vi "溶解氧电极校准.vi"() -> ()   [LabVIEW 2016, in "斯坦道多参数.lvlib"]
uses:
  <vilib>/Utility/miscctls.llb/LVPointTypeDef.ctl
  <vilib>/Analysis/NI_AALBase.lvlib
panel:
  out "标液2":string="饱和标准液"
  out "标液1":string="零点标准液"
  in  "刷新按钮":bool
  out "第二点信号值":dbl
  out "第一点信号值":dbl
  out "通讯状态":string
  out "第二点校准值":dbl
  out "第一点校准值":dbl
  out "最小值":sgl format="%#.2f"
  out "最大值":sgl format="%#.2f"
  in  "校准模式":u16(ring)=1 items=["两点校准", "单点校准"]
  in  "校准停止":bool
  in  "校准启动":bool
  out "波形图表":dbl(graph) caption="历史曲线"
  out "变异系数":dbl format="%#.6f"
  out "standard deviation":dbl caption="标准差" format="%#.2f"
  out "mean":dbl caption="均值" format="%#.2f"
  out "测量读值":dbl caption="测量值" format="%#.2f"
  out "偏移值补偿":dbl caption="溶解氧偏移修正值" format="%#.2f"
  out "饱和度值":dbl format="%#.2f"
  out "提示":string
  out "气压补偿值":dbl format="%#.2f"
  out "盐度补偿值":dbl format="%#.2f"
  out "电极斜率":dbl format="%#.6f"
  out "电极零点":dbl format="%#.6f"
  # "溶解氧电极设定"
  # "%"
  # "%"
  # "ppt"
  # "hPa"
  # "请选择校准模式:"
  # "mg/L"
  # "%"
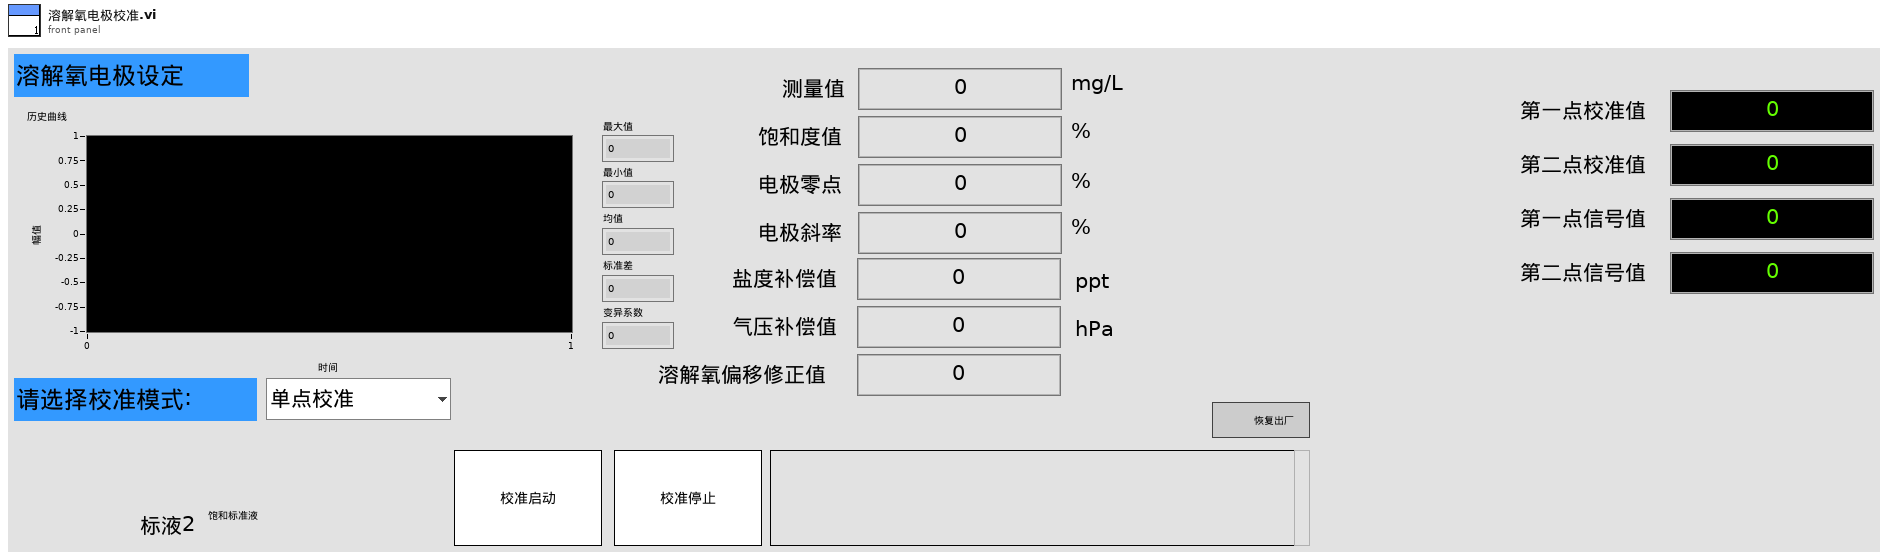
[diagram p1: front panel]
types:
  T1 = typedef "LVPointTypeDef.ctl" = cluster{"Horizontal":i16, "Vertical":i16}
  T2 = cluster{"电极状态标志":u16, "电极型号标志":u16, "溶解氧测量值":sgl, "温度测量值":sgl, "溶解氧饱和度值":sgl, "盐度补偿值":sgl, "大气压补偿值":sgl, "溶解氧偏移修正值":sgl, "温度偏移修正值":sgl, "手动温度补偿值":sgl, "溶解氧电极零点":sgl, "溶解氧电极斜率":sgl, "第1点标准值记录":sgl, "第1点信号值记录":sgl, "第1点温度值记录":sgl, "第2点标准值记录":sgl, "第2点信号值记录":sgl, "第2点温度值记录":sgl, "命令滤波设定":u16, "温度模式":enum16{"ATC", "MTC"}, "生产批次":u16, "电极序号":u16, "串口地址":u16, "串口波特率":enum16{"9600", "19200", "115200"}, "串口校验位":enum16{"NONE", "ODD", "EVEN"}, "串口停止位":enum16{"1bit", "2bit"}, "第一点标准值":sgl, "第二点标准值":sgl}
  T3 = enum8{"Enabled", "Disabled", "Disabled and Grayed Out"}
  T4 = cluster{"ph":bool, "DO":bool, "Cond":bool, "Turb":bool, "叶绿素a":bool, "藻密度":bool, "ORP":bool}
  T5 = cluster{"温度测量值":sgl, "测量值":sgl, "温度偏移修正值":sgl, "信号值":sgl}
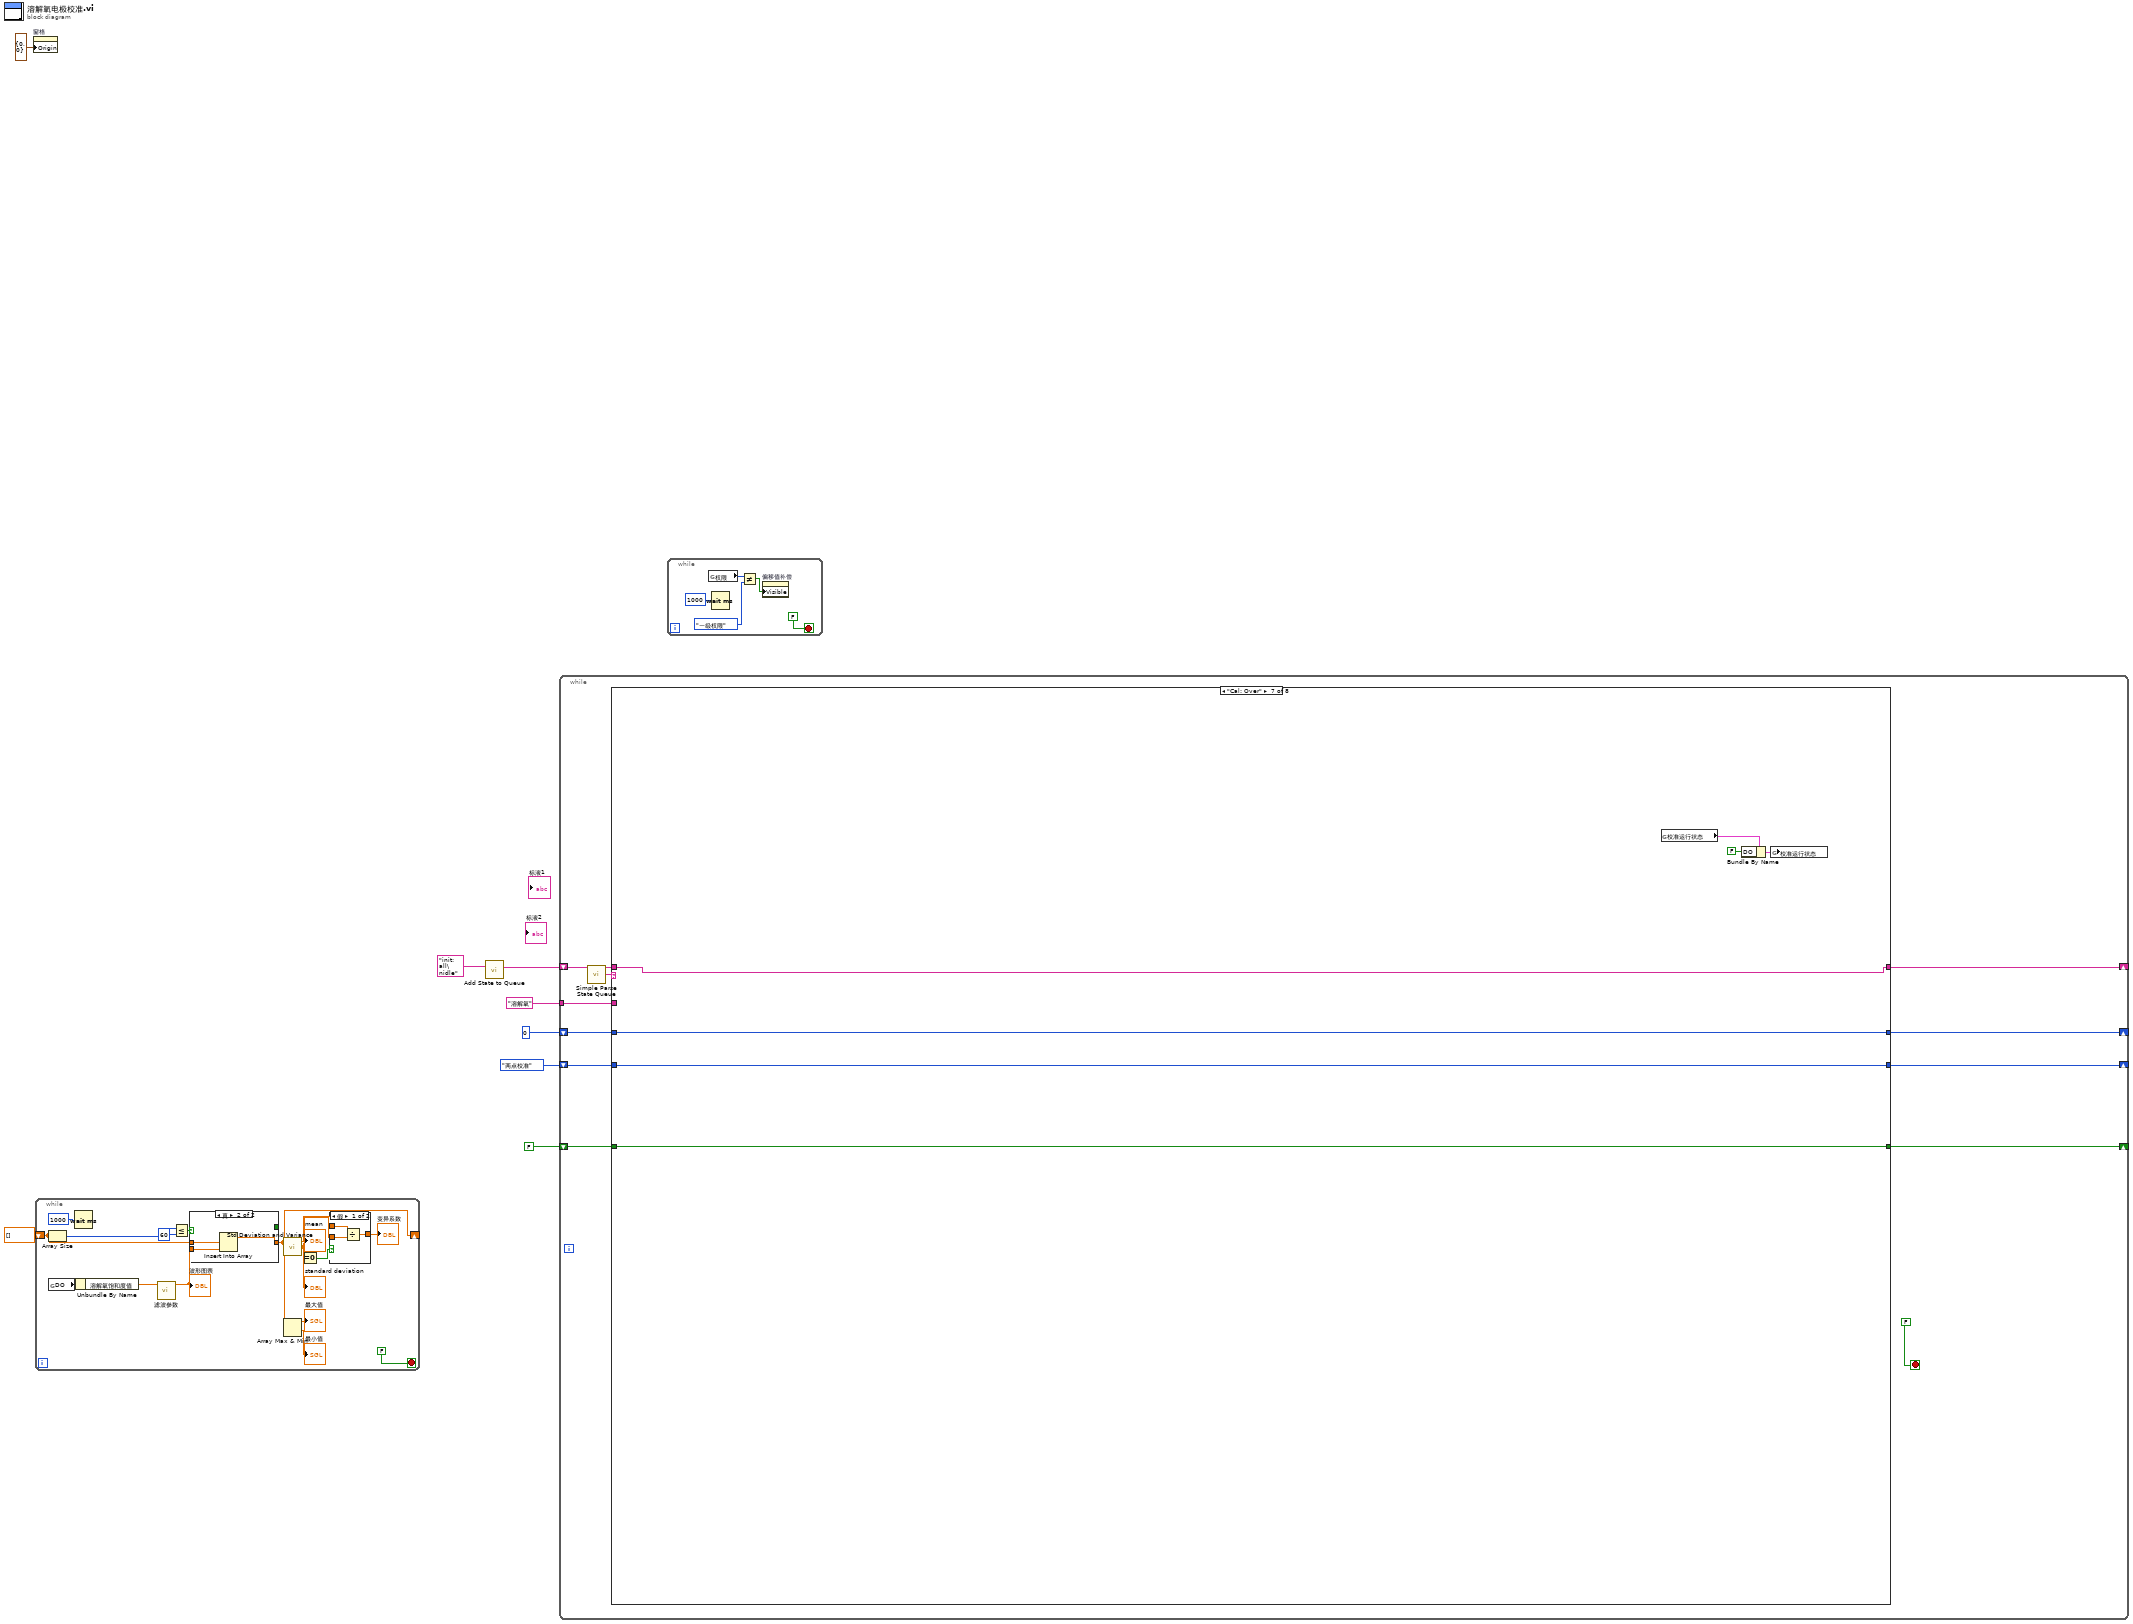
[diagram p0: block diagram]
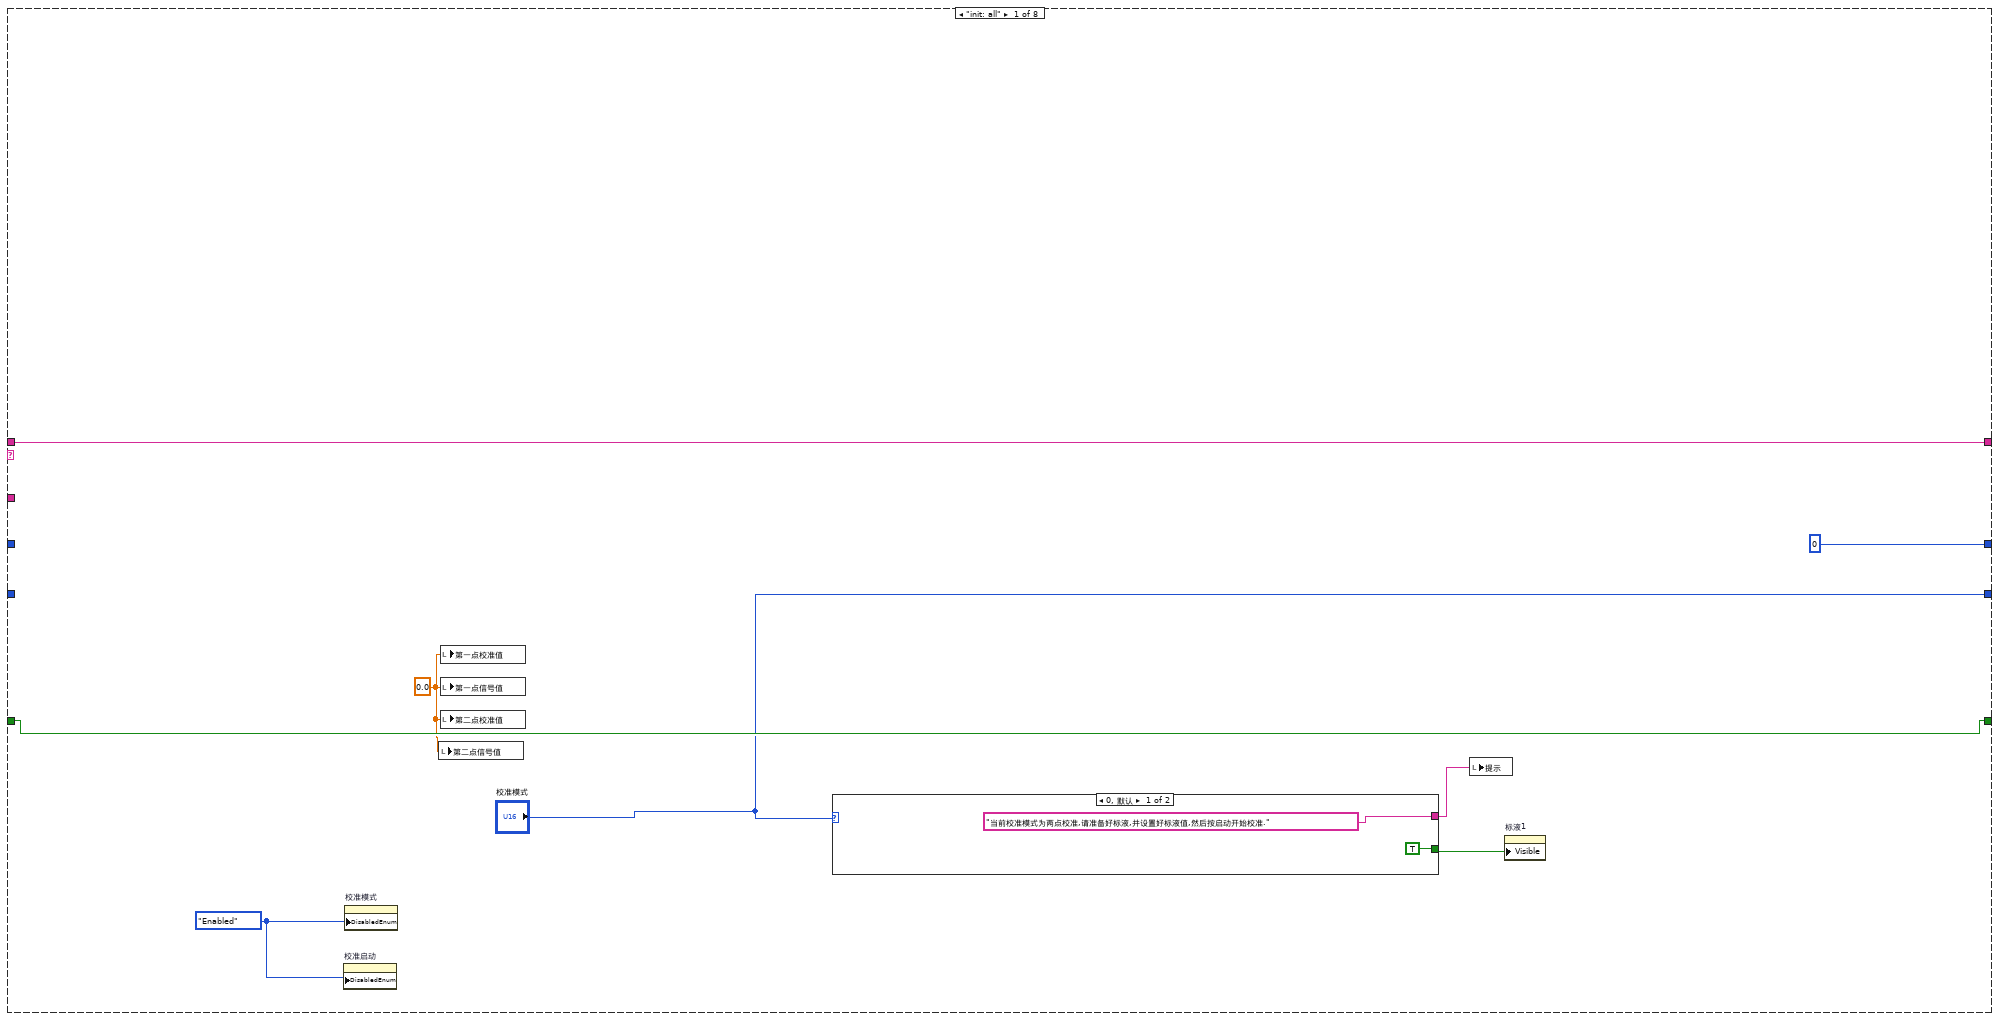
[diagram p2: hidden frame]
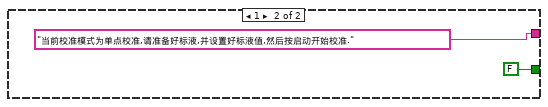
[diagram p3: hidden frame]
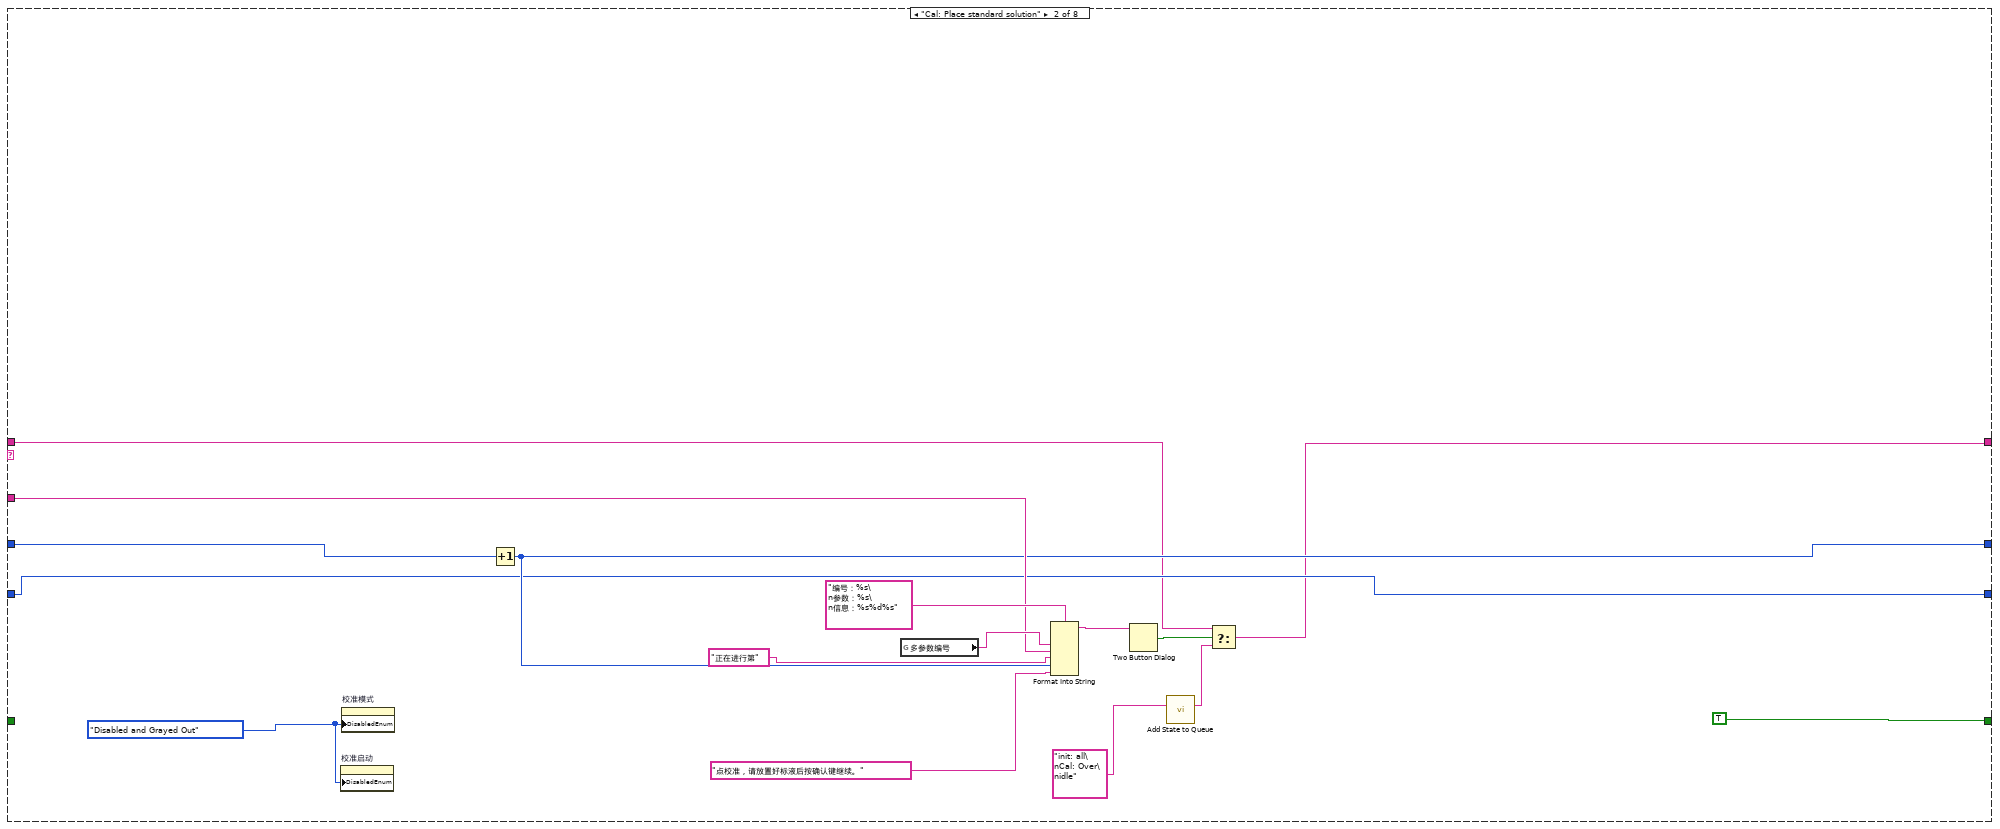
[diagram p4: hidden frame]
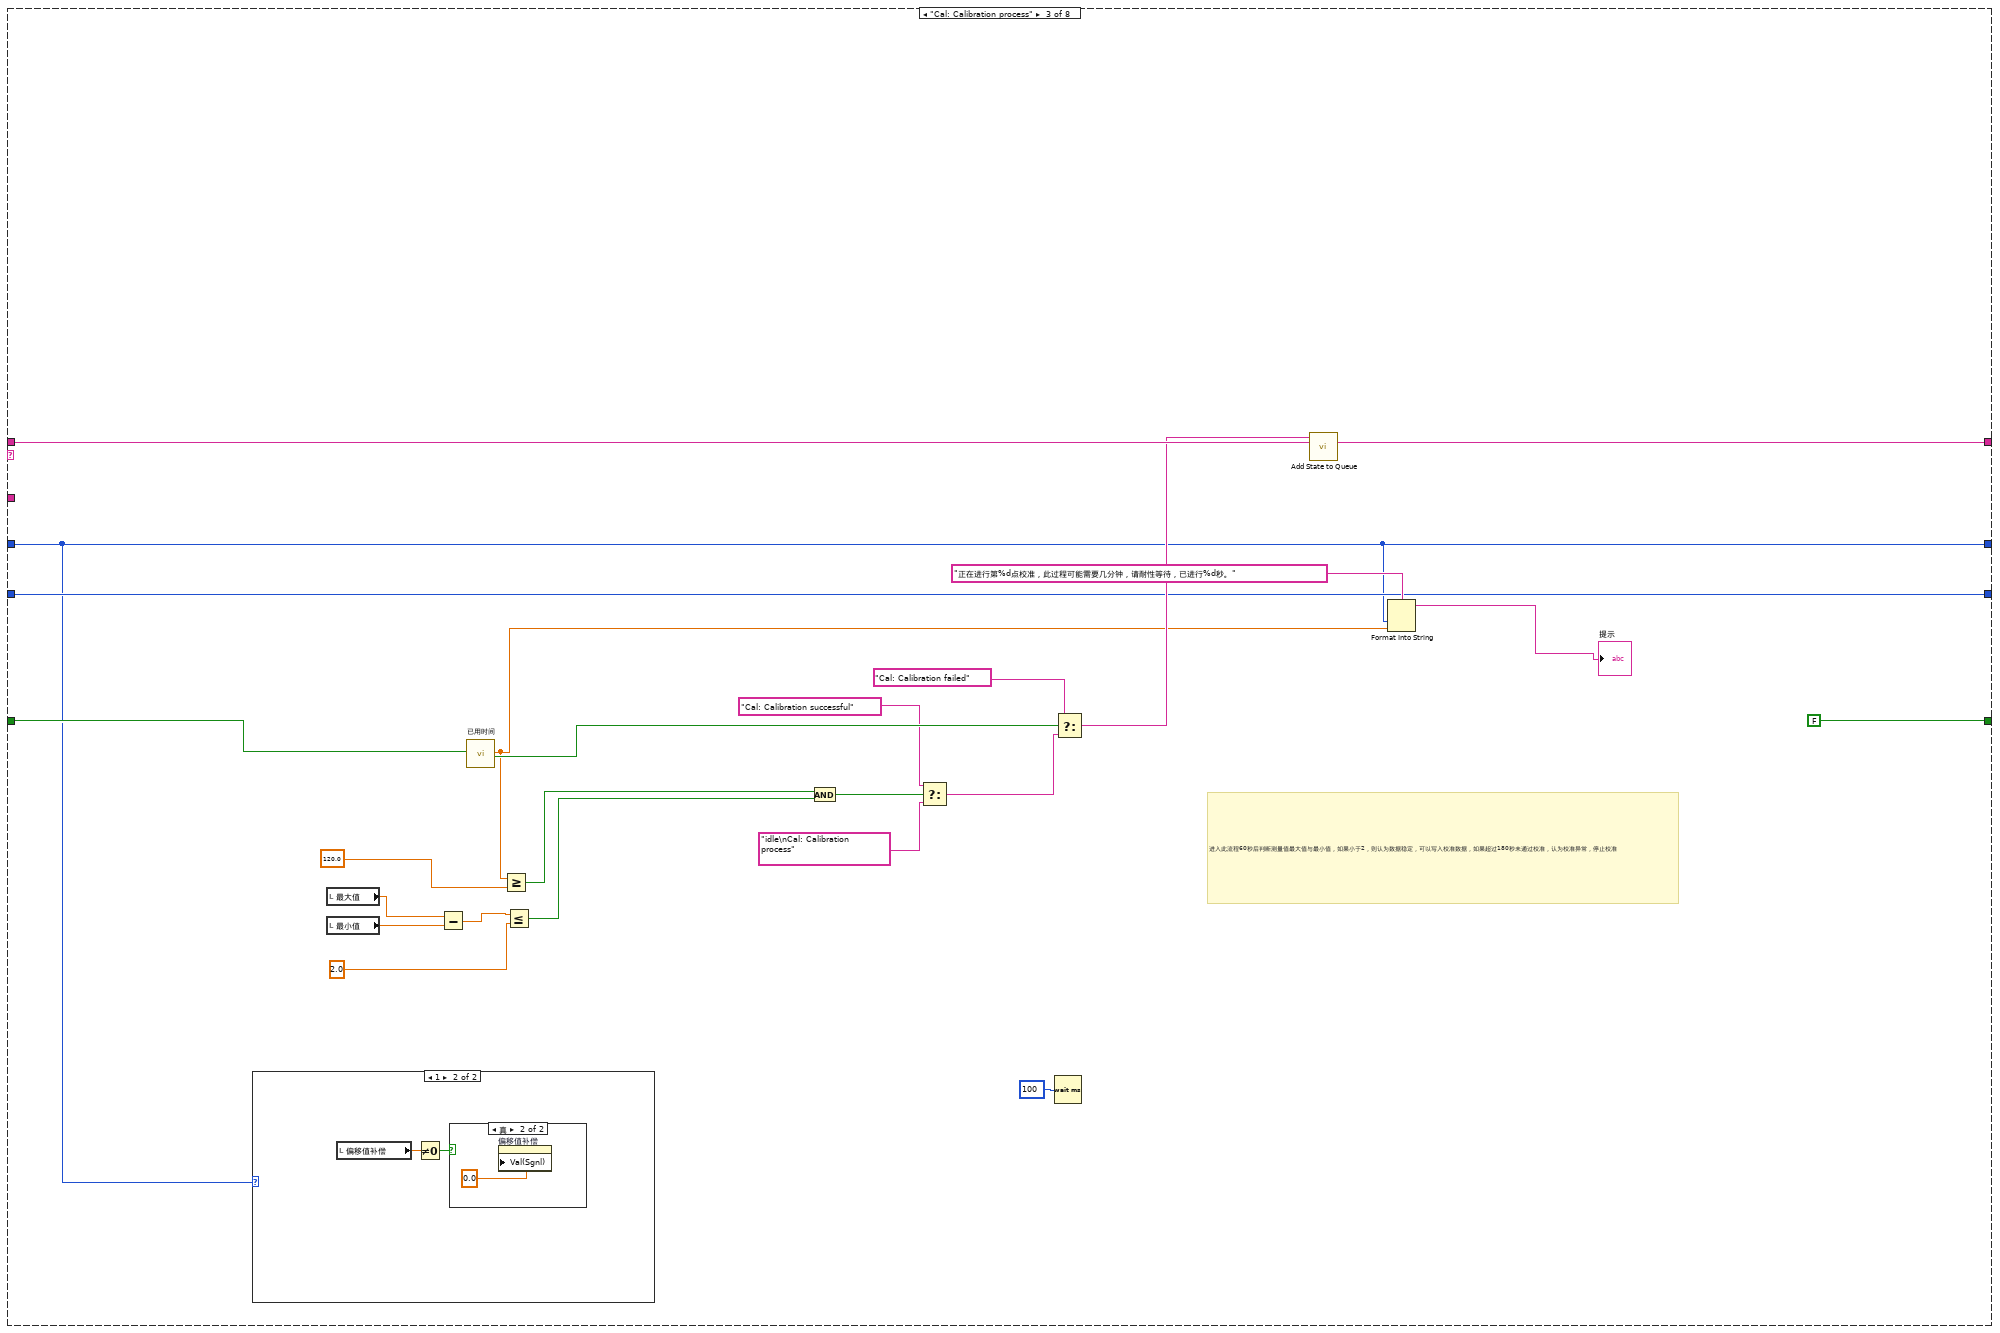
[diagram p5: hidden frame]
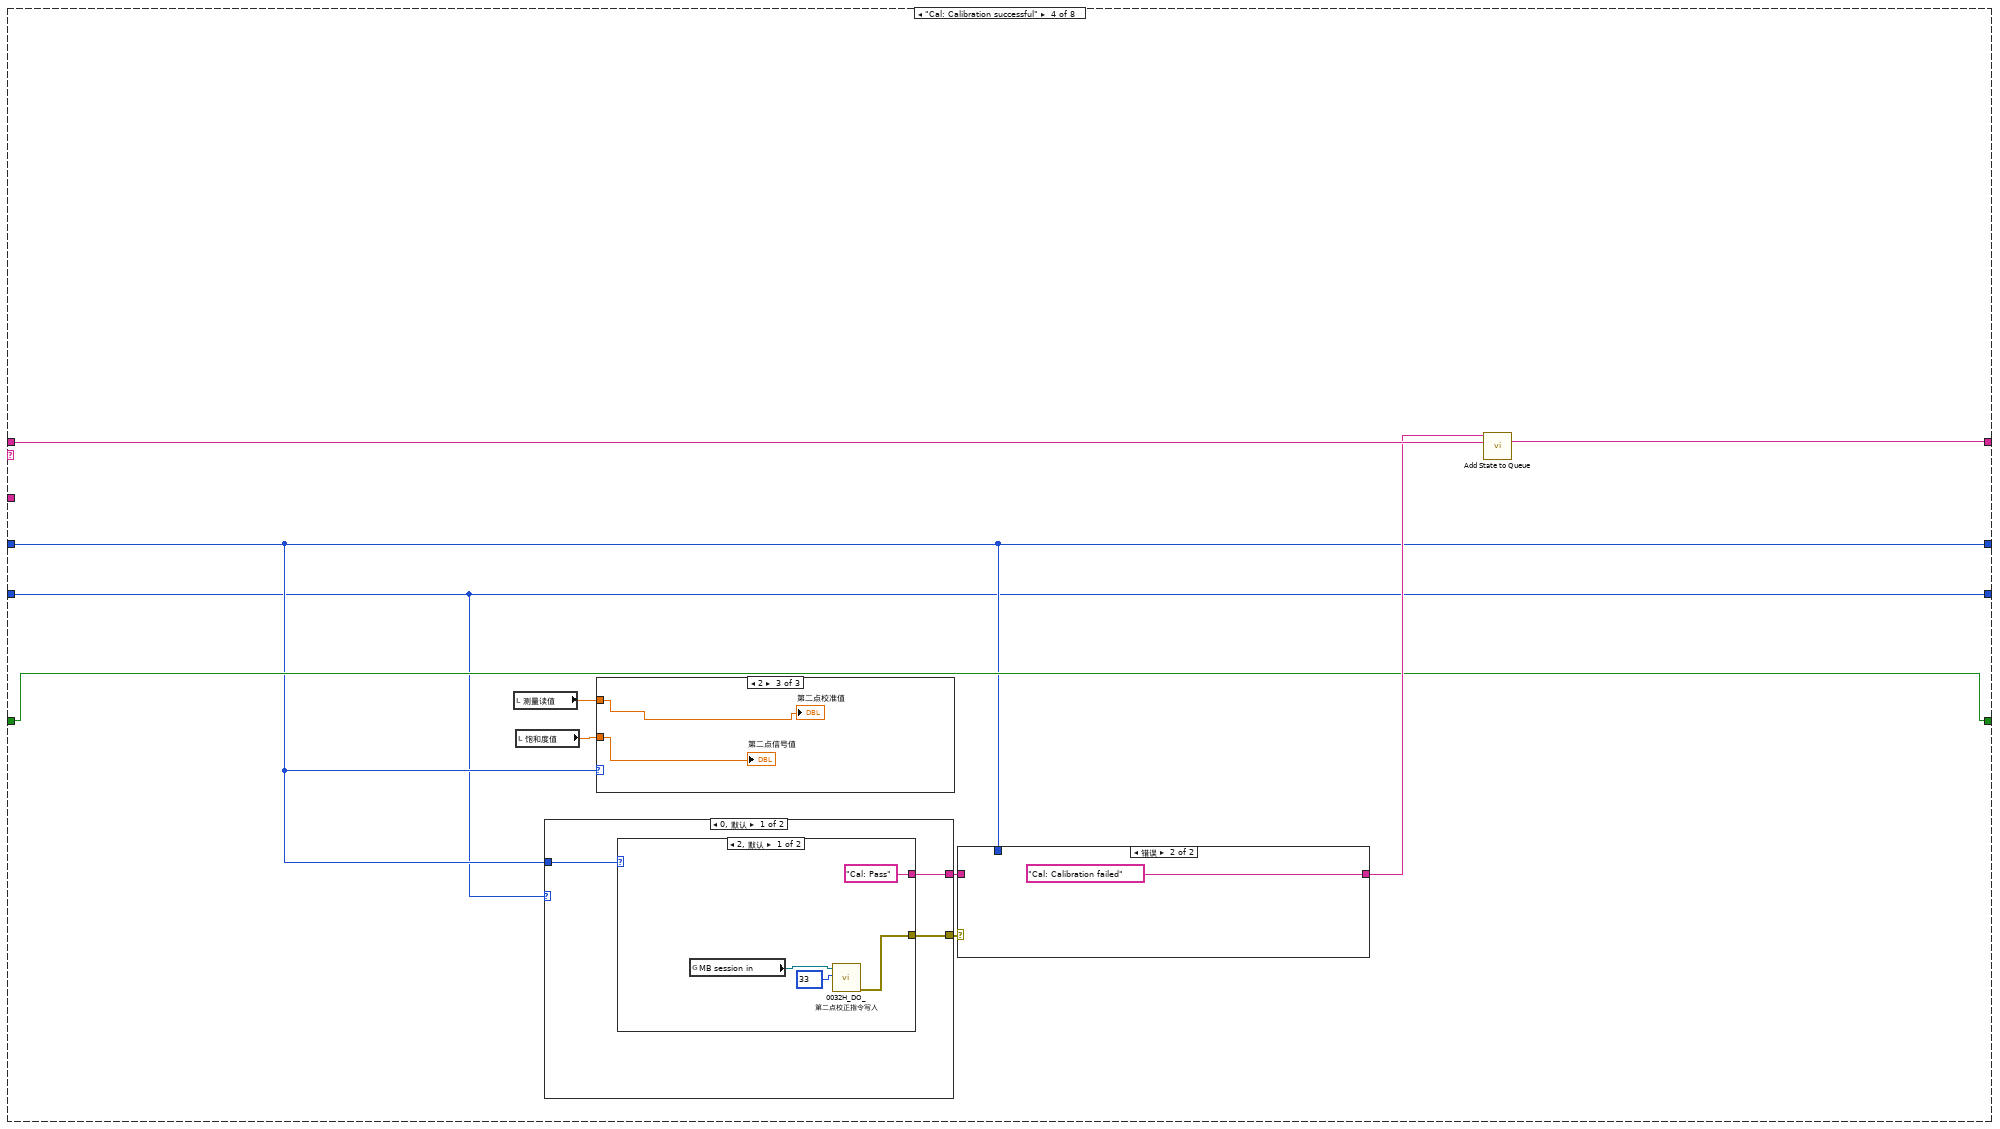
[diagram p8: hidden frame]
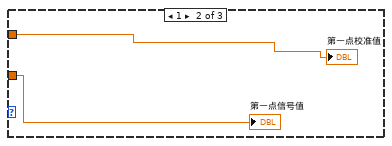
[diagram p10: hidden frame]
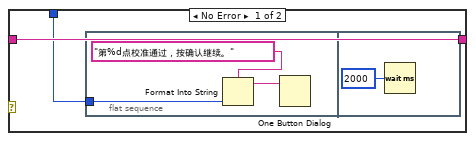
[diagram p11: hidden frame]
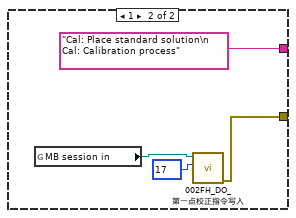
[diagram p12: hidden frame]
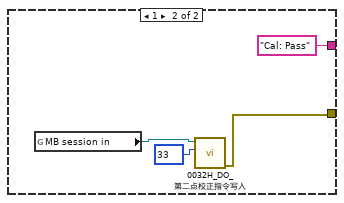
[diagram p13: hidden frame]
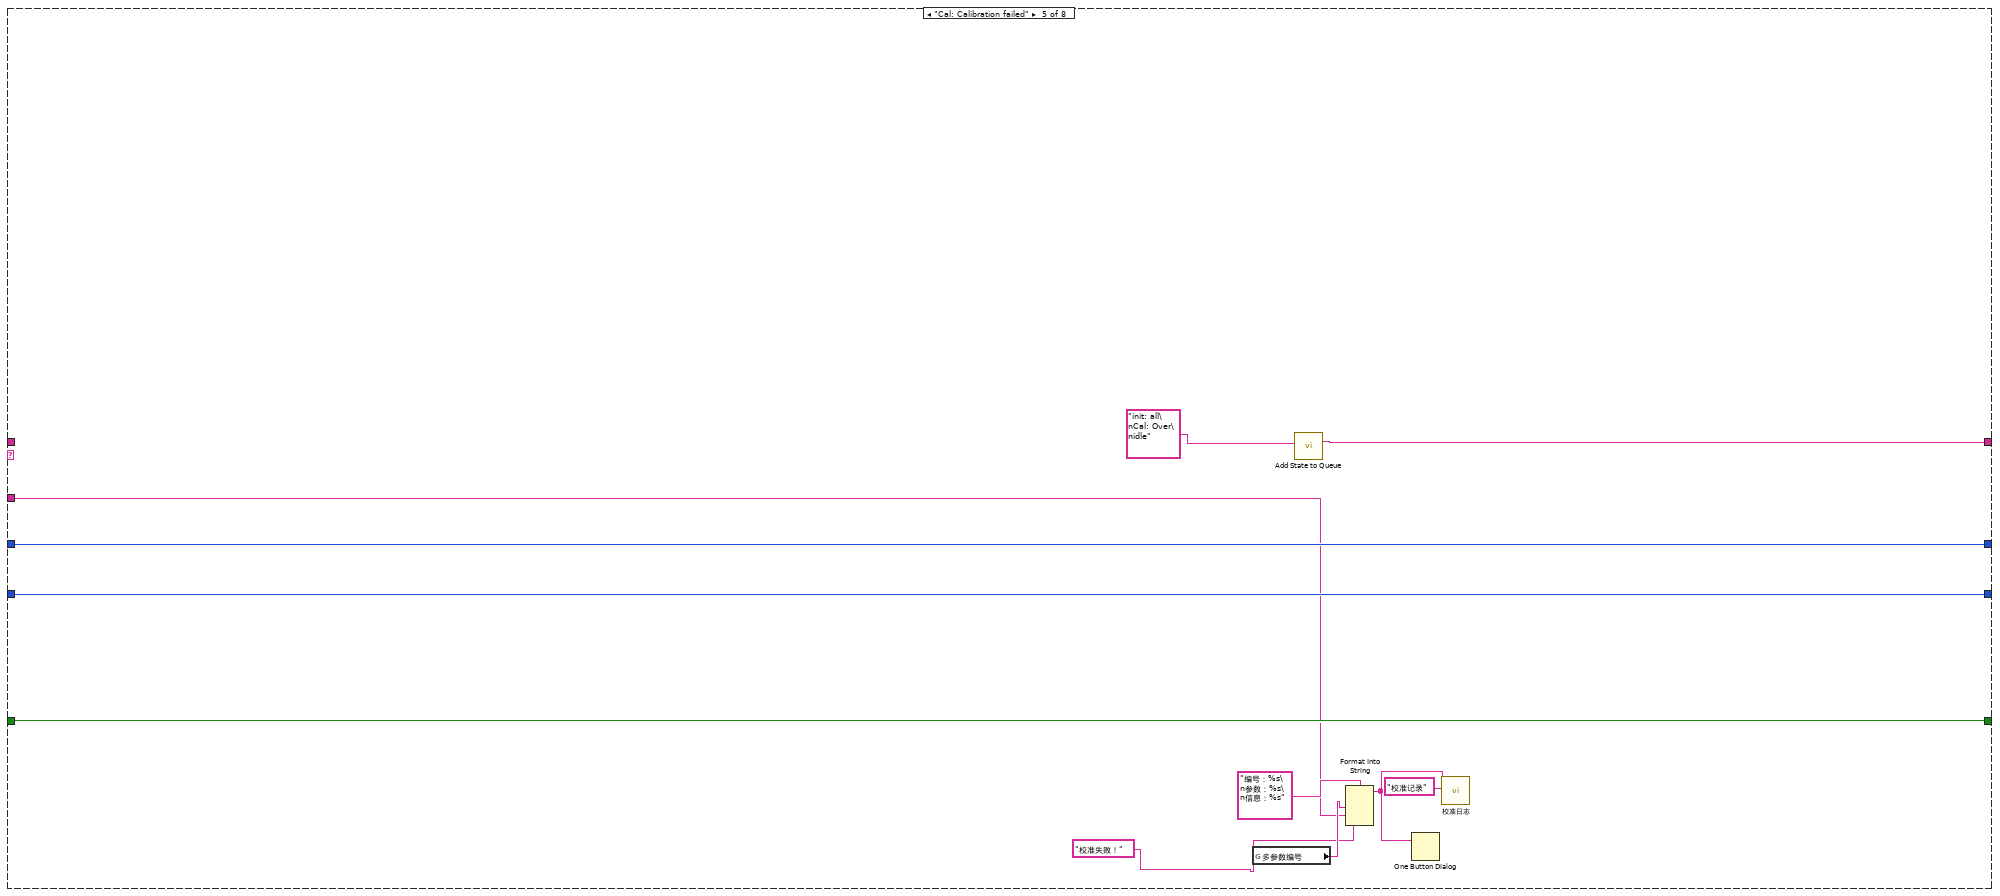
[diagram p14: hidden frame]
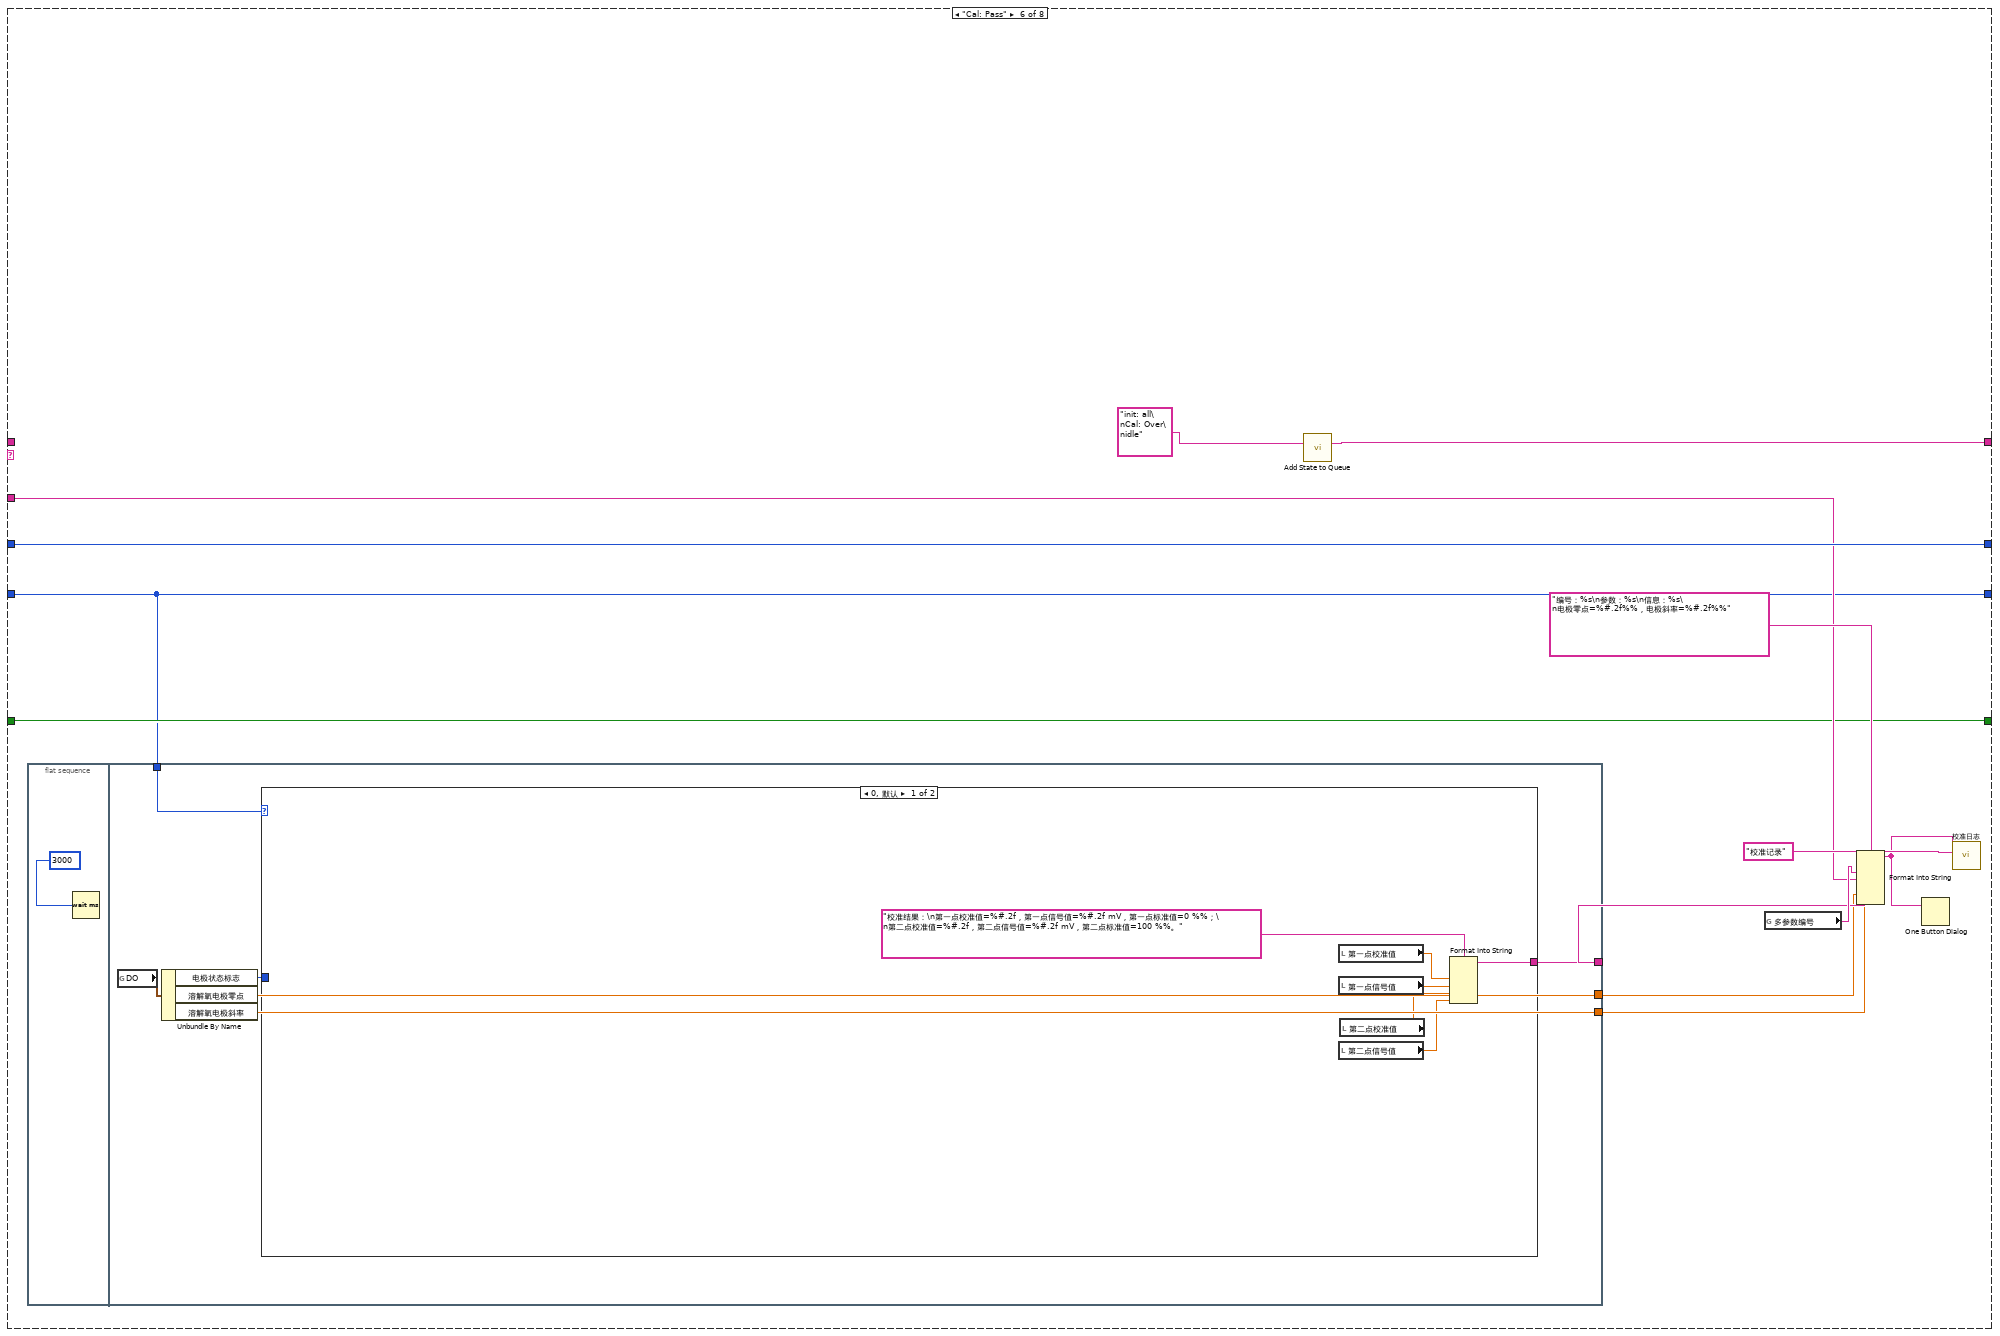
[diagram p15: hidden frame]
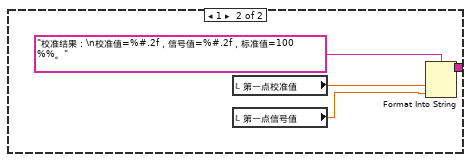
[diagram p16: hidden frame]
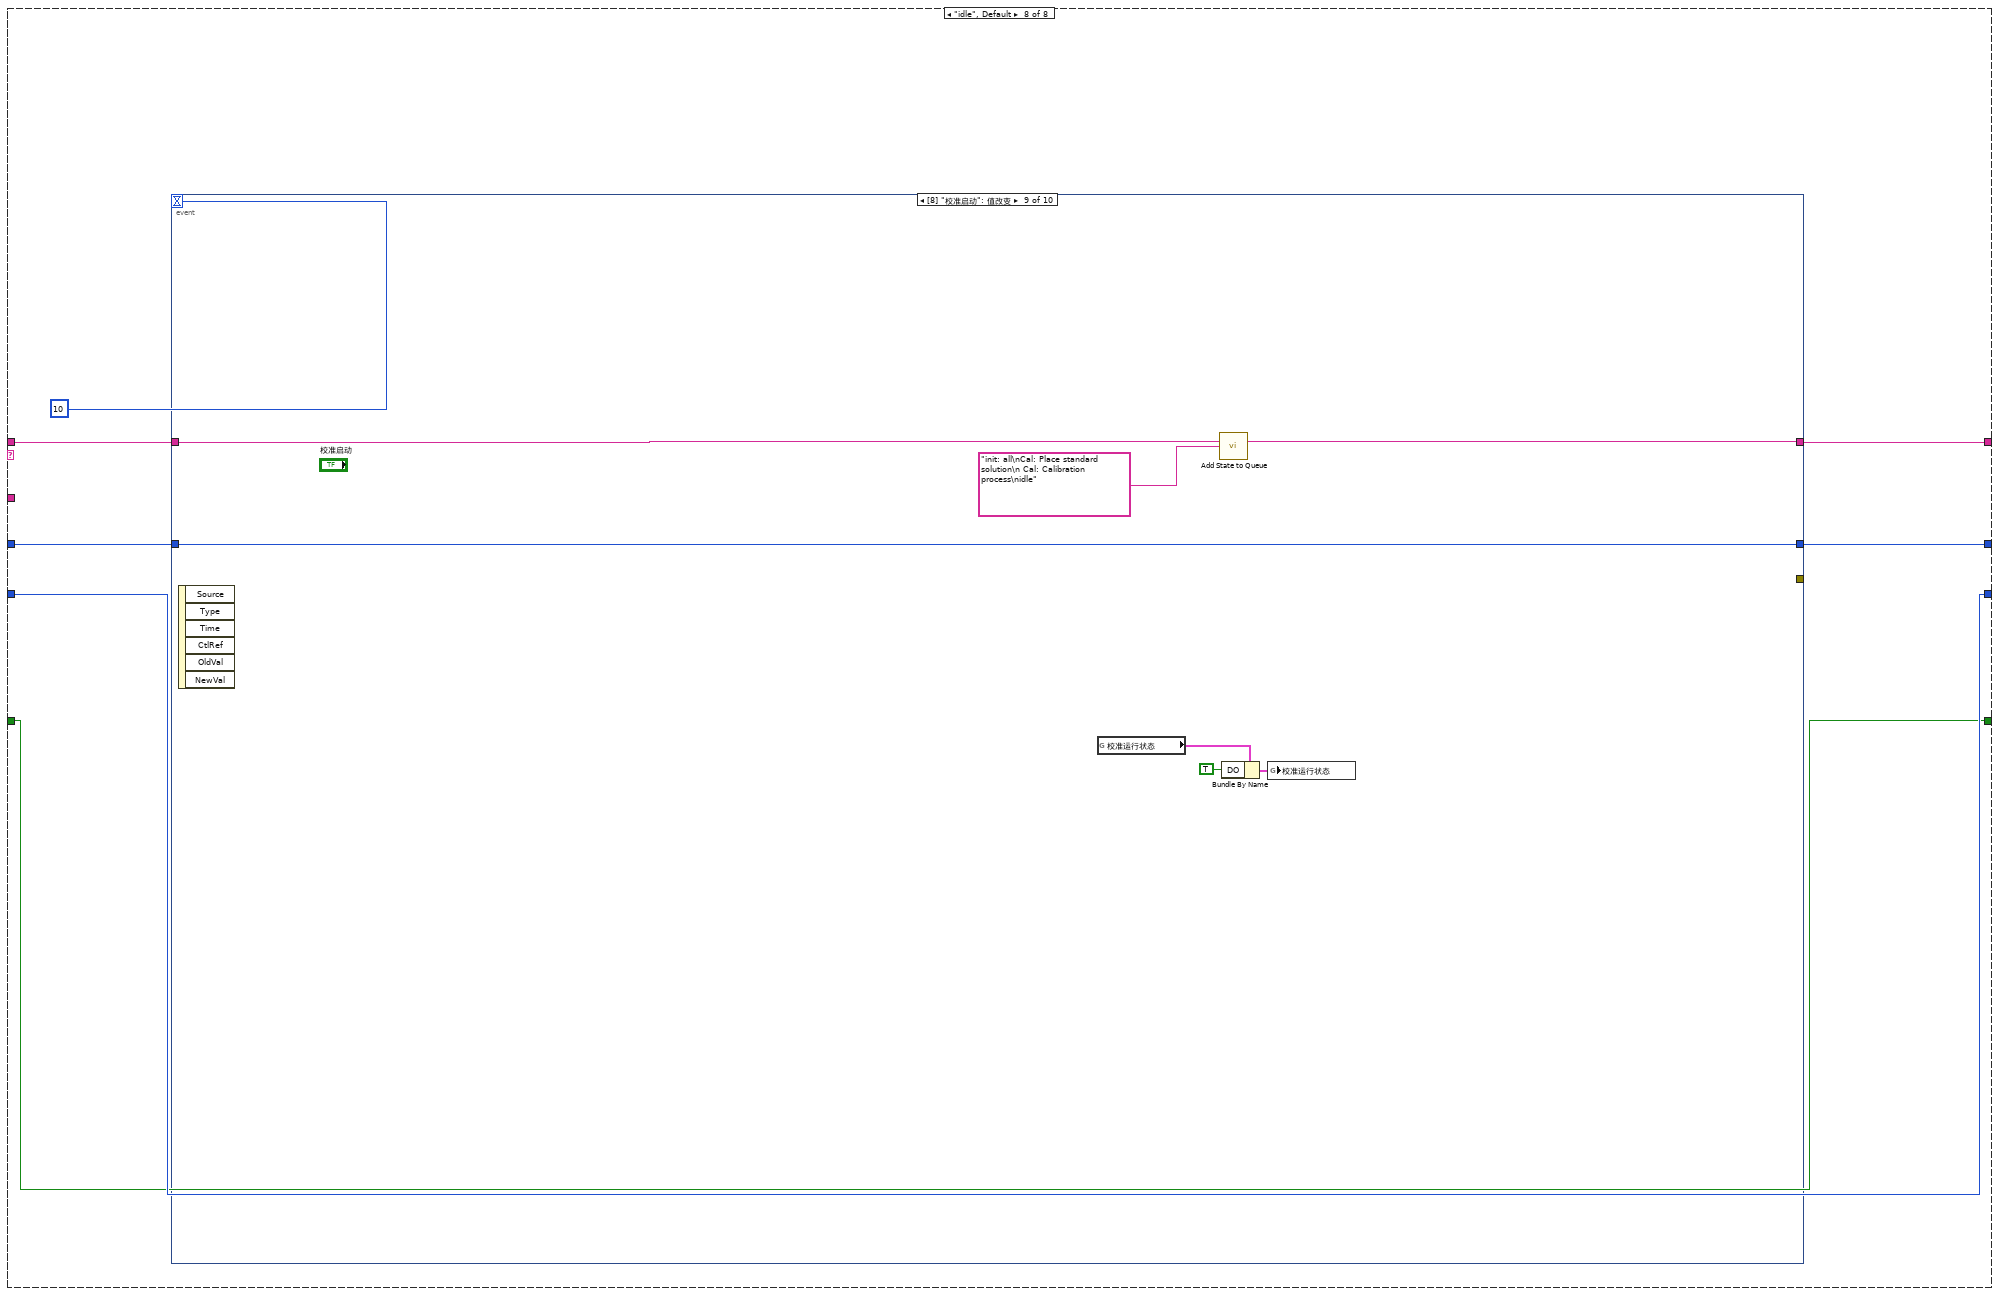
[diagram p17: hidden frame]
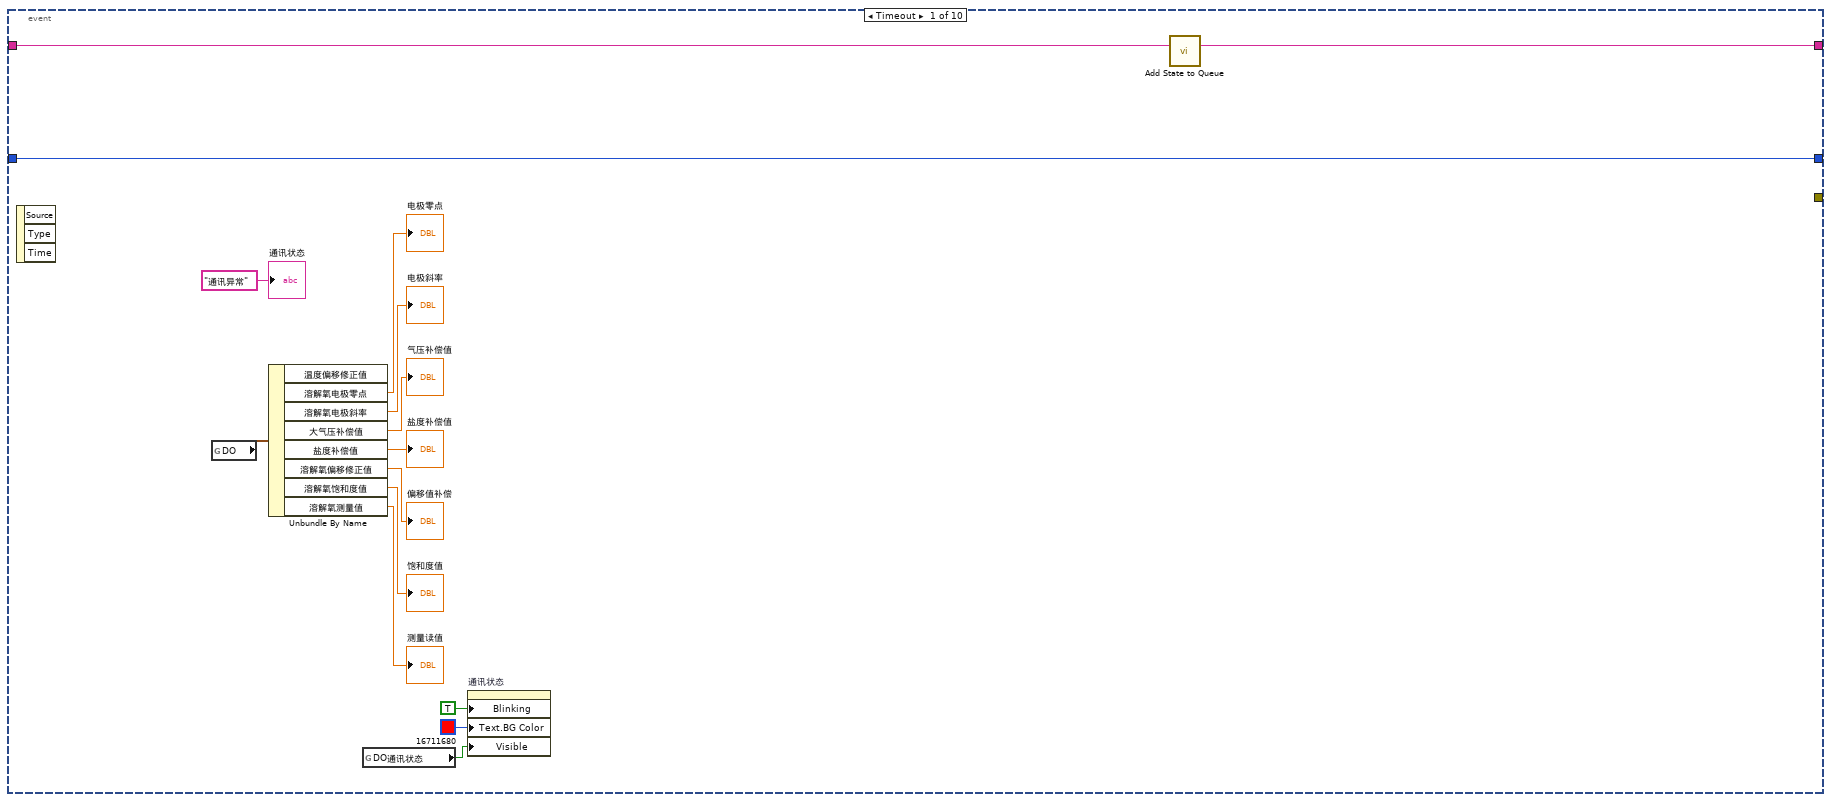
[diagram p18: hidden frame]
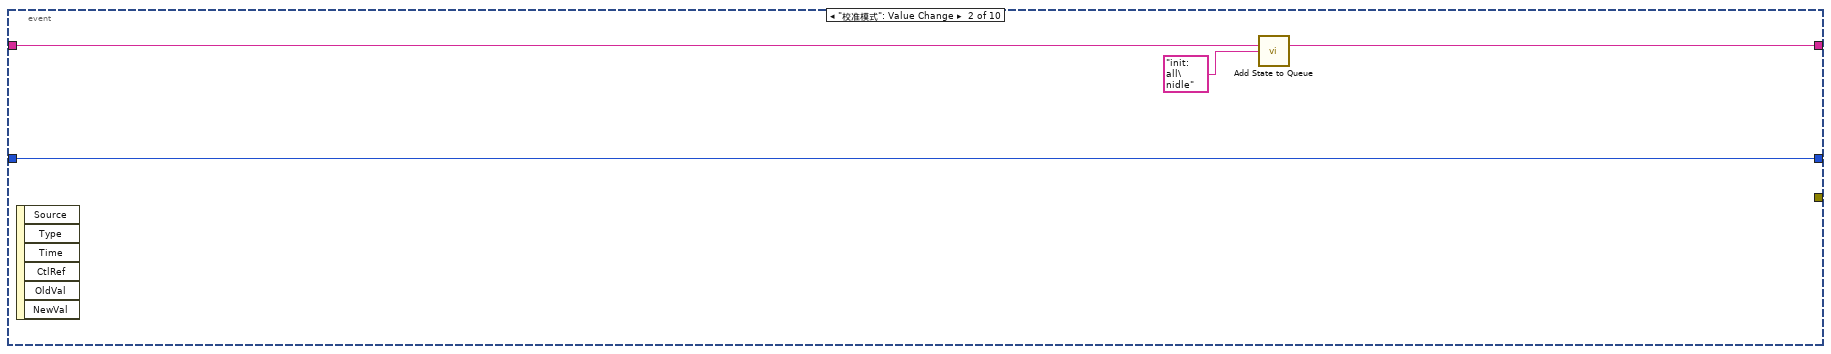
[diagram p19: hidden frame]
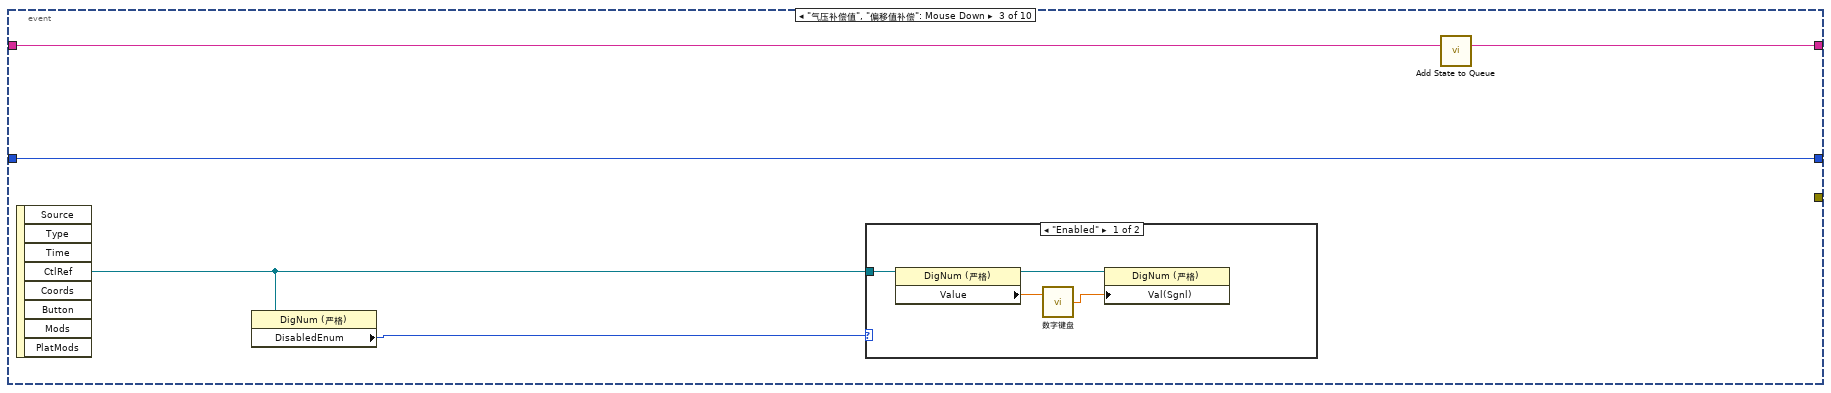
[diagram p20: hidden frame]
diagram:
  n1 = property on="窗格" class="Pane"("Origin"=T1 {"Horizontal"=0, "Vertical"=0} ("原点")) -> ()  [unwired: 2 in, 2 out]
  n2 = while {
    shift-right: [w13] -> _
    shift-left: sgl[] [] -> [w20]
    stop <- FALSE stop-if-true
    n3 = Array Size(array=w20) -> (size(s)=w22:i32)
    n4 = global read "国弘过程全局变量.vi" "DO"() -> (w16:T2)
    n5 = Wait (ms)(milliseconds to wait=u32 1000 ("等待时间（毫秒）")) -> ()  [unwired: 1 out]
    n6 = Unbundle By Name(w16) -> ("溶解氧饱和度值"=w10:sgl)
    n7 = call "滤波参数.vi"("x"=w10) -> ("mode"=w9:dbl)  [unwired: 10 in]
    "波形图表" <- w9
    n8 = Less Or Equal?(x=w22, y=60) -> (x <= y?=w21:bool)
    n9 = case shown="真" w21 {
      tunnel: w20 -> [w33 w36]
      tunnel: w9 -> [w31 w35]
      tunnel: [w29 w34] -> w13
      tunnel: [TRUE _] -> _
      frame False {
        n10 = Replace Array Subset(array=w33, new element=w31) -> (w32:sgl[])  [unwired: 1 in]
        n11 = Rotate 1D Array(1:w32, 2:-1 ("n")) -> (0:w29:sgl[])
      }
      frame True {
        n12 = Insert Into Array(array=w36, new element=w35) -> (w34:sgl[])  [unwired: 1 in]
      }
    }
    n13 = call <vilib>:"Std Deviation and Variance.vi"("X"=w13) -> ("mean"=w15:dbl, "standard deviation"=w14:dbl)  [unwired: 1 in, 1 out]
    "mean" <- w15
    "standard deviation" <- w14
    n14 = Array Max & Min(array=w13) -> (max value=→"最大值":sgl, min value=→"最小值":sgl)  [unwired: 2 out]
    n15 = Equal To 0?(x=w15) -> (x = 0?=w19:bool)
    n16 = case shown="假" w19 {
      tunnel: w14 -> [w27 _]
      tunnel: [w26 _] -> w18
      tunnel: w15 -> [w25 _]
      frame False {
        n17 = Divide(x=w27, y=w25) -> (x/y=w26:dbl)
      }
      frame True {
      }
    }
    "变异系数" <- w18
  }
  n18 = call "Add State to Queue.vi"("State(s) In (\"\")"="init: all\nidle" ("State(s) In (\"\")")) -> ("States Out"=w5:string)  [unwired: 14 in]
  n19 = while {
    shift-right: [w44] -> _
    shift-left: w5 -> [w48]
    shift-right: [w41] -> _
    shift-left: 0 -> [w43]
    tunnel: "溶解氧" ("State(s) In (\"\")") -> [w42]
    shift-right: [w39] -> _
    shift-left: enum16{"两点校准", "单点校准"}."两点校准" ("校准模式") -> [w40]
    shift-right: [w37] -> _
    shift-left: FALSE -> [w38]
    stop <- FALSE stop-if-true
    n20 = call "Simple Parse State Queue.vi"("State Queue"=w48) -> ("Remain States"=w45:string, "Next State"=w46:string)  [unwired: 13 in]
    n21 = case shown="\"Cal: Over\"" w46 {
      tunnel: w45 -> [w56 w64 w95 w111 _ _ w187 w194]
      tunnel: [w56 w63 w94 w110 w147 w154 w187 w193] -> w44
      tunnel: w43 -> [_ w72 w79 w105 w150 w163 w186 w191]
      tunnel: w42 -> [_ w73 _ _ w141 w159 _ _]
      tunnel: [0 w70 w79 w105 w150 w163 w186 w192] -> w41
      tunnel: w40 -> [_ w69 w80 w104 w149 w155 w185 w190]
      tunnel: ["校准模式" w69 w80 w104 w149 w155 w185 w190] -> w39
      tunnel: w38 -> [w53 _ w82 w106 w148 w158 w184 w188]
      tunnel: [w53 TRUE FALSE w106 w148 w158 w184 w188] -> w37
      frame "init: all" {
        w51 = T3."Enabled" ("禁用")
        w52 = 0.0 ("第一点校准值")
        n22 = property on="校准启动" class="Bool"("DisabledEnum"=w51) -> ()  [unwired: 2 in, 2 out]
        n23 = property on="校准模式" class="Ring (严格)"("DisabledEnum"=w51) -> ()  [unwired: 2 in, 2 out]
        n24 = local write "第二点信号值"(w52) -> ()
        n25 = local write "第一点校准值"(w52) -> ()
        n26 = local write "第一点信号值"(w52) -> ()
        n27 = local write "第二点校准值"(w52) -> ()
        n28 = case shown="0, 默认" "校准模式" {
          tunnel: ["当前校准模式为两点校准,请准备好标液,并设置好标液值,然后按启动开始校准." ("提示") "当前校准模式为单点校准,请准备好标液,并设置好标液值,然后按启动开始校准." ("提示")] -> w55
          tunnel: [TRUE ("可见") FALSE ("可见")] -> w49
          frame 0, Default {
          }
          frame 1 {
          }
        }
        n29 = local write "提示"(w55) -> ()
        n30 = property on="标液1" class="Str"("Visible"=w49) -> ()  [unwired: 2 in, 2 out]
      }
      frame "Cal: Place standard solution" {
        w62 = T3."Disabled and Grayed Out" ("禁用")
        n31 = property on="校准启动" class="Bool"("DisabledEnum"=w62) -> ()  [unwired: 2 in, 2 out]
        n32 = property on="校准模式" class="Ring (严格)"("DisabledEnum"=w62) -> ()  [unwired: 2 in, 2 out]
        n33 = Increment(x=w72) -> (x+1=w70:i32)
        n34 = global read "多参数全局变量.vi" "多参数编号"() -> (w75:string)
        n35 = Format Into String(format string="编号：%s\n参数：%s\n信息：%s%d%s" ("格式字符串"), w75, w73, "正在进行第" ("消息"), w70, "点校准，请放置好标液后按确认键继续。" ("消息")) -> (resulting string=w67:string)  [unwired: 2 in, 1 out]
        n36 = Two Button Dialog(message=w67) -> (T button?=w66:bool)  [unwired: 2 in]
        n37 = call "Add State to Queue.vi"("State(s) In (\"\")"="init: all\nCal: Over\nidle" ("State(s) In (\"\")")) -> ("States Out"=w65:string)  [unwired: 14 in]
        n38 = Select(t=w64, s=w66, f=w65) -> (s? t:f=w63:string)
      }
      frame "Cal: Calibration process" {
        # "进入此流程60秒后判断测量值最大值与最小值，如果小于2，则认为数据稳定，可以写入校准数据，如果超过180秒未通过校准，认为校准异常，停止校准"
        n39 = case shown="1" w79 {
          frame 0, Default {
          }
          frame 1 {
            n40 = local read "偏移值补偿"() -> (w101:dbl)
            n41 = Not Equal To 0?(x=w101) -> (x != 0?=w102:bool)
            n42 = case shown="真" w102 {
              frame False {
              }
              frame True {
                n43 = property on="偏移值补偿" class="DigNum (严格)"("Val(Sgnl)"=0.0 ("值(信号)")) -> ()  [unwired: 2 in, 2 out]
              }
            }
          }
        }
        n44 = local read "最大值"() -> (w99:sgl)
        n45 = local read "最小值"() -> (w98:sgl)
        n46 = Subtract(x=w99, y=w98) -> (x-y=w100:sgl)
        n47 = call "已用时间"("Reset"=w82) -> ("Elapsed Time (s)"=w78:dbl, "Time has Elapsed"=w96:bool)  [unwired: 11 in, 6 out]
        n48 = Greater Or Equal?(x=w78, y=120.0) -> (x >= y?=w91:bool)
        n49 = Less Or Equal?(x=w100, y=2.0) -> (x <= y?=w87:bool)
        n50 = And(x=w91, y=w87) -> (x .and. y?=w88:bool)
        n51 = Select(t="Cal: Calibration successful" ("State(s) In (\"\")"), s=w88, f="idle\nCal: Calibration process" ("State(s) In (\"\")")) -> (s? t:f=w86:string)
        n52 = Wait (ms)(milliseconds to wait=u32 100 ("等待时间（毫秒）")) -> ()  [unwired: 1 out]
        n53 = Select(t="Cal: Calibration failed" ("State(s) In (\"\")"), s=w96, f=w86) -> (s? t:f=w85:string)
        n54 = call "Add State to Queue.vi"("State(s) In Front (\"\")"=w85, "State(s) In (\"\")"=w95) -> ("States Out"=w94:string)  [unwired: 13 in]
        n55 = Format Into String(format string="正在进行第%d点校准，此过程可能需要几分钟，请耐性等待，已进行%d秒。" ("格式字符串"), w79, w78) -> (resulting string=→"提示":string)  [unwired: 2 in, 1 out]
      }
      frame "Cal: Calibration successful" {
        n56 = local read "测量读值"() -> (w107:dbl)
        n57 = local read "饱和度值"() -> (w108:dbl)
        n58 = case shown="0, 默认" w104 {
          tunnel: [w127 w136] -> w113
          tunnel: [w126 "Cal: Pass" ("State(s) In (\"\")")] -> w112
          tunnel: w105 -> [w125 _]
          frame 0, Default {
            n59 = case shown="2, 默认" w125 {
              tunnel: [w128 w132] -> w127
              tunnel: ["Cal: Pass" ("State(s) In (\"\")") "Cal: Place standard solution\n Cal: Calibration process" ("State(s) In (\"\")")] -> w126
              frame 2, Default {
                n60 = global read "多参数全局变量.vi" "MB session in"() -> (w129:refnum<class "MB_Master.lvclass">)
                n61 = call "0032H_DO_第二点校正指令写入.vi"("数值"=u16 33, "MB session in"=w129) -> ("error out"=w128:errorcluster)  [unwired: 8 in, 1 out]
              }
              frame 1 {
                n62 = global read "多参数全局变量.vi" "MB session in"() -> (w133:refnum<class "MB_Master.lvclass">)
                n63 = call "002FH_DO_第一点校正指令写入.vi"("数值"=u16 17, "MB session in"=w133) -> ("error out"=w132:errorcluster)  [unwired: 8 in, 1 out]
              }
            }
          }
          frame 1 {
            n64 = global read "多参数全局变量.vi" "MB session in"() -> (w138:refnum<class "MB_Master.lvclass">)
            n65 = call "0032H_DO_第二点校正指令写入.vi"("数值"=u16 33, "MB session in"=w138) -> ("error out"=w136:errorcluster)  [unwired: 8 in, 1 out]
          }
        }
        n66 = case shown="2" w105 {
          tunnel: w108 -> [_ w115 w117]
          tunnel: w107 -> [_ w114 w116]
          frame 0, Default {
          }
          frame 1 {
            "第一点信号值" <- w115
            "第一点校准值" <- w114
          }
          frame 2 {
            "第二点信号值" <- w117
            "第二点校准值" <- w116
          }
        }
        n67 = case shown="错误" w113 {
          tunnel: w112 -> [w119 _]
          tunnel: [w119 "Cal: Calibration failed" ("State(s) In (\"\")")] -> w109
          tunnel: w105 -> [w118 _]
          frame No Error {
            n68 = flat-sequence {
              tunnel: w118 -> [w120]
              frame #0 {
                n69 = Format Into String(format string="第%d点校准通过，按确认继续。" ("格式字符串"), w120) -> (resulting string=w122:string)  [unwired: 2 in, 1 out]
                n70 = One Button Dialog(message=w122) -> ()  [unwired: 1 in, 1 out]
              }
              frame #1 {
                n71 = Wait (ms)(milliseconds to wait=u32 2000 ("等待时间（毫秒）")) -> ()  [unwired: 1 out]
              }
            }
          }
          frame Error {
          }
        }
        n72 = call "Add State to Queue.vi"("State(s) In Front (\"\")"=w109, "State(s) In (\"\")"=w111) -> ("States Out"=w110:string)  [unwired: 13 in]
      }
      frame "Cal: Calibration failed" {
        n73 = global read "多参数全局变量.vi" "多参数编号"() -> (w144:string)
        n74 = call "Add State to Queue.vi"("State(s) In (\"\")"="init: all\nCal: Over\nidle" ("State(s) In (\"\")")) -> ("States Out"=w147:string)  [unwired: 14 in]
        n75 = Format Into String(format string="编号：%s\n参数：%s\n信息：%s" ("格式字符串"), w144, w141, "校准失败！" ("消息")) -> (resulting string=w143:string)  [unwired: 2 in, 1 out]
        n76 = One Button Dialog(message=w143) -> ()  [unwired: 1 in, 1 out]
        n77 = call "校准日志.vi"("table"="校准记录", "日志信息"=w143) -> ()  [unwired: 9 in, 1 out]
      }
      frame "Cal: Pass" {
        n78 = flat-sequence {
          tunnel: [w168] -> w156
          tunnel: w155 -> [w167]
          tunnel: [w166] -> w153
          tunnel: [w165] -> w152
          frame #0 {
            n79 = Wait (ms)(milliseconds to wait=u32 3000 ("等待时间（毫秒）")) -> ()  [unwired: 1 out]
          }
          frame #1 {
            n80 = global read "国弘过程全局变量.vi" "DO"() -> (w169:T2)
            n81 = Unbundle By Name(w169) -> ("电极状态标志"=w170:u16, "溶解氧电极零点"=w166:sgl, "溶解氧电极斜率"=w165:sgl)
            n82 = case shown="0, 默认" w167 {
              tunnel: [w176 w180] -> w168
              tunnel: w170 -> [_ _]
              frame 0, Default {
                n83 = local read "第一点校准值"() -> (w174:dbl)
                n84 = local read "第一点信号值"() -> (w175:dbl)
                n85 = local read "第二点信号值"() -> (w171:dbl)
                n86 = local read "第二点校准值"() -> (w172:dbl)
                n87 = Format Into String(format string="校准结果：\n第一点校准值=%#.2f，第一点信号值=%#.2f mV，第一点标准值=0 %%；\n第二点校准值=%#.2f，第二点信号值=%#.2f mV，第二点标准值=100 %%。" ("提示"), w174, w175, w172, w171) -> (resulting string=w176:string)  [unwired: 2 in, 1 out]
              }
              frame 1 {
                n88 = local read "第一点校准值"() -> (w179:dbl)
                n89 = local read "第一点信号值"() -> (w177:dbl)
                n90 = Format Into String(format string="校准结果：\n校准值=%#.2f，信号值=%#.2f，标准值=100 %%。" ("提示"), w179, w177) -> (resulting string=w180:string)  [unwired: 2 in, 1 out]
              }
            }
          }
        }
        n91 = call "Add State to Queue.vi"("State(s) In (\"\")"="init: all\nCal: Over\nidle" ("State(s) In (\"\")")) -> ("States Out"=w154:string)  [unwired: 14 in]
        n92 = global read "多参数全局变量.vi" "多参数编号"() -> (w160:string)
        n93 = Format Into String(format string="编号：%s\n参数：%s\n信息：%s\n电极零点=%#.2f%%，电极斜率=%#.2f%%" ("格式字符串"), w160, w159, w156, w153, w152) -> (resulting string=w157:string)  [unwired: 2 in, 1 out]
        n94 = One Button Dialog(message=w157) -> ()  [unwired: 1 in, 1 out]
        n95 = call "校准日志.vi"("table"="校准记录", "日志信息"=w157) -> ()  [unwired: 9 in, 1 out]
      }
      frame "Cal: Over" {
        n96 = global read "多参数全局变量.vi" "校准运行状态"() -> (w182:T4)
        n97 = Bundle By Name(cluster=w182, "DO"=FALSE) -> (w183:T4)
        n98 = global write "多参数全局变量.vi" "校准运行状态"(w183) -> ()
      }
      frame "idle", Default {
        n99 = event shown="[8] \"校准启动\": 值改变" {
          selector: _ -> [_ _ _ _ _ _ _ _ _ _]
          dyn-events: _ -> [_ _ _ _ _ _ _ _ _ _]
          timeout: 10 -> [_ _ _ _ _ _ _ _ _ _]
          tunnel: [_ _ _ _ w240 w246 w252 _ _ _] -> _
          tunnel: w194 -> [w209 w213 w216 w225 w239 w245 w251 w259 w270 _]
          tunnel: [w208 w212 w217 w226 w243 w249 w255 w258 w269 w272] -> w193
          tunnel: [w207 w210 w218 w227 w244 w250 w256 w257 w267 w273] -> w192
          tunnel: w191 -> [w207 w210 w218 w227 w244 w250 w256 w257 w267 w273]
          event Timeout {
            n100 = event-data() -> ()  [unwired: 1 in, 3 out]
            n101 = global read "国弘过程全局变量.vi" "DO"() -> (w195:T2)
            n102 = Unbundle By Name(w195) -> ("溶解氧电极零点"=→"电极零点":sgl, "溶解氧电极斜率"=→"电极斜率":sgl, "大气压补偿值"=→"气压补偿值":sgl, "盐度补偿值"=→"盐度补偿值":sgl, "溶解氧偏移修正值"=→"偏移值补偿":sgl, "溶解氧饱和度值"=→"饱和度值":sgl, "溶解氧测量值"=→"测量读值":sgl)  [unwired: 1 out]
            n103 = global read "多参数全局变量.vi" "DO通讯状态"() -> (w206:bool)
            n104 = property on="通讯状态" class="Str"("Blinking"=TRUE ("闪烁"), "Text.BG Color"=u32 16711680, "Visible"=w206) -> ()  [unwired: 2 in, 2 out]
            n105 = call "Add State to Queue.vi"("State(s) In (\"\")"=w209) -> ("States Out"=w208:string)  [unwired: 14 in]
            "通讯状态" <- "通讯异常" ("当前串口")
          }
          event "校准模式": Value Change {
            n106 = event-data() -> ()  [unwired: 1 in, 6 out]
            n107 = call "Add State to Queue.vi"("State(s) In (\"\")"=w213, "State(s) At Back (\"\")"="init: all\nidle" ("State(s) In (\"\")")) -> ("States Out"=w212:string)  [unwired: 13 in]
          }
          event "气压补偿值", "偏移值补偿": Mouse Down {
            n108 = event-data() -> ("CtlRef"=w215:refnum<vi>)  [unwired: 1 in, 7 out]
            n109 = property class="DigNum (严格)"(reference=w215) -> ("DisabledEnum"=w214:T3)  [unwired: 1 in, 2 out]
            n110 = case shown="\"Enabled\"" w214 {
              tunnel: w215 -> [w222 _]
              frame "Enabled" {
                n111 = property class="DigNum (严格)"(reference=w222) -> (reference out=w219:refnum<vi>, "Value"=w220:dbl)  [unwired: 1 in, 1 out]
                n112 = call "数字键盘.vi"("OldNumber"=w220) -> ("NewNumber"=w221:dbl)  [unwired: 1 in]
                n113 = property class="DigNum (严格)"(reference=w219, "Val(Sgnl)"=w221) -> ()  [unwired: 1 in, 2 out]
              }
              frame "Disabled", Default {
              }
            }
            n114 = call "Add State to Queue.vi"("State(s) In (\"\")"=w216) -> ("States Out"=w217:string)  [unwired: 14 in]
          }
          event "盐度补偿值": Mouse Down {
            n115 = event-data() -> ("CtlRef"=w224:refnum<vi>)  [unwired: 1 in, 7 out]
            n116 = property class="DigNum (严格)"(reference=w224) -> ("DisabledEnum"=w223:T3)  [unwired: 1 in, 2 out]
            n117 = case shown="\"Enabled\"" w223 {
              tunnel: w224 -> [w236 _]
              frame "Enabled" {
                n118 = global read "断电保存变量.vi" "Cond"() -> (w228:bool)
                n119 = case shown="真" w228 {
                  tunnel: [_ w237] -> w233
                  frame False {
                  }
                  frame True {
                    n120 = Two Button Dialog(message="是否使用系统测试值自动补偿" ("消息")) -> (T button?=w237:bool)  [unwired: 2 in]
                  }
                }
                n121 = global read "多参数全局变量.vi" "盐度显示"() -> (w232:T5)
                n122 = Unbundle By Name(w232) -> ("测量值"=w231:sgl)
                n123 = property class="DigNum (严格)"(reference=w236) -> (reference out=w234:refnum<vi>, "Value"=w230:dbl)  [unwired: 1 in, 1 out]
                n124 = Select(t=w231, s=w233, f=w230) -> (s? t:f=w229:dbl)
                n125 = call "数字键盘.vi"("OldNumber"=w229) -> ("NewNumber"=w235:dbl)  [unwired: 1 in]
                n126 = property class="DigNum (严格)"(reference=w234, "Val(Sgnl)"=w235) -> ()  [unwired: 1 in, 2 out]
              }
              frame "Disabled", Default {
              }
            }
            n127 = call "Add State to Queue.vi"("State(s) In (\"\")"=w225) -> ("States Out"=w226:string)  [unwired: 14 in]
          }
          event "盐度补偿值": Value Change {
            n128 = event-data() -> ("NewVal"=w241:dbl)  [unwired: 1 in, 5 out]
            n129 = global read "多参数全局变量.vi" "MB session in"() -> (w242:refnum<class "MB_Master.lvclass">)
            n130 = call "0008H_DO_盐度补偿值写入.vi"("数值"=w241, "MB session in"=w242) -> ("error out"=w240:errorcluster)  [unwired: 8 in, 1 out]
            n131 = call "Add State to Queue.vi"("State(s) In (\"\")"=w239) -> ("States Out"=w243:string)  [unwired: 14 in]
          }
          event "气压补偿值": Value Change {
            n132 = event-data() -> ("NewVal"=w247:dbl)  [unwired: 1 in, 5 out]
            n133 = global read "多参数全局变量.vi" "MB session in"() -> (w248:refnum<class "MB_Master.lvclass">)
            n134 = call "000AH_DO_大气压补偿值写入.vi"("数值"=w247, "MB session in"=w248) -> ("error out"=w246:errorcluster)  [unwired: 8 in, 1 out]
            n135 = call "Add State to Queue.vi"("State(s) In (\"\")"=w245) -> ("States Out"=w249:string)  [unwired: 14 in]
          }
          event "偏移值补偿": Value Change {
            n136 = event-data() -> ("NewVal"=w253:dbl)  [unwired: 1 in, 5 out]
            n137 = global read "多参数全局变量.vi" "MB session in"() -> (w254:refnum<class "MB_Master.lvclass">)
            n138 = call "000CH_DO_DO偏移修正值写入.vi"("数值"=w253, "MB session in"=w254) -> ("error out"=w252:errorcluster)  [unwired: 8 in, 1 out]
            n139 = call "Add State to Queue.vi"("State(s) In (\"\")"=w251) -> ("States Out"=w255:string)  [unwired: 14 in]
          }
          event "刷新按钮": Value Change {
            n140 = event-data() -> ()  [unwired: 1 in, 6 out]
            n141 = call "Add State to Queue.vi"("State(s) In (\"\")"=w259) -> ("States Out"=w258:string)  [unwired: 14 in]
            n142 = Two Button Dialog(message="请再次确实是否恢复出厂设置！" ("消息")) -> (T button?=w261:bool)  [unwired: 2 in]
            n143 = case shown="真" w261 {
              frame False {
              }
              frame True {
                w262 = u16 33 items=["Factory Reset"=33] ("数值")
                n144 = global read "多参数全局变量.vi" "MB session in"() -> (w263:refnum<class "MB_Master.lvclass">)
                n145 = call "0026H_DO_命令寄存器写入.vi"("数值"=w262, "MB session in"=w263) -> ()  [unwired: 8 in, 2 out]
              }
            }
          }
          event "校准启动": Value Change {
            n146 = event-data() -> ()  [unwired: 1 in, 6 out]
            n147 = global read "多参数全局变量.vi" "校准运行状态"() -> (w265:T4)
            n148 = call "Add State to Queue.vi"("State(s) In (\"\")"=w270, "State(s) At Back (\"\")"="init: all\nCal: Place standard solution\n Cal: Calibration process\nidle" ("State(s) In (\"\")")) -> ("States Out"=w269:string)  [unwired: 13 in]
            n149 = Bundle By Name(cluster=w265, "DO"=TRUE) -> (w266:T4)
            n150 = global write "多参数全局变量.vi" "校准运行状态"(w266) -> ()
          }
          event "校准停止": Value Change {
            n151 = event-data() -> ()  [unwired: 1 in, 6 out]
            n152 = call "Add State to Queue.vi"("State(s) In (\"\")"="init: all\nCal: Over\nidle" ("State(s) In (\"\")")) -> ("States Out"=w272:string)  [unwired: 14 in]
          }
        }
      }
    }
  }
  n153 = while {
    stop <- FALSE stop-if-true
    n154 = global read "多参数全局变量.vi" "权限"() -> (w277:enum16{"一级权限", "二级权限", "三级权限"})
    n155 = Wait (ms)(milliseconds to wait=u32 1000 ("等待时间（毫秒）")) -> ()  [unwired: 1 out]
    n156 = Not Equal?(x=w277, y=enum16{"一级权限", "二级权限", "三级权限"}."一级权限") -> (x != y?=w275:bool)
    n157 = property on="偏移值补偿" class="DigNum (严格)"("Visible"=w275) -> ()  [unwired: 2 in, 2 out]
  }
